vi "Simulation Kobuki Sensors.vi"(8 "error in":errorcluster, 9 "Feedback Input":T1, 10 "Robot":T2, 11 "simulator":T8={"configuration"={"maxTime"=5.0, "enableVisualization"=TRUE, "Environment Definition"=path "simulation configuration.ini", "Record Location"=path "Simulation Record.xml", "autograde?"=TRUE, "interactive?"=FALSE, "Feedback Mode"=enum."debug navigation", "Robot State Charts"=[path "C:/Users/blueuser/Desktop/Robo Sim Berkley/cpsgrader-release-0.4/Simulators/EECS149lab/src/LabVIEW/statechart/Simulation Statechart.vi"], "statechart"=path "iRobot Navigation State Machine.vi"}, "Statechart\ndisplay"=refnum, "first step?"=FALSE, "Robots Simulation Statecharts"=[], "Robots"=[]}) -> (0 "error out":errorcluster, 1 "Feedback Output":T1, 2 "sensors":T3 {"Kobuki Sensors"."Charger Source" items=["DISCHARGING"=0, "DOCKING_CHARGED"=2, "DOCKING_CHARGING"=6, "ADAPTER_CHARGED"=18, "ADAPTER_CHARGING"=22]; "accelerometer"."z axis (g)" format="%.3f"; "accelerometer"."y axis (g)" format="%.3f"; "accelerometer"."x axis (g)" format="%.3f"}, 3 "simulator":T8={"configuration"={"maxTime"=5.0, "enableVisualization"=TRUE, "Environment Definition"=path "simulation configuration.ini", "Record Location"=path "Simulation Record.xml", "autograde?"=TRUE, "interactive?"=FALSE, "Feedback Mode"=enum."debug navigation", "Robot State Charts"=[path "C:/Users/blueuser/Desktop/Robo Sim Berkley/cpsgrader-release-0.4/Simulators/EECS149lab/src/LabVIEW/statechart/Simulation Statechart.vi"], "statechart"=path "iRobot Navigation State Machine.vi"}, "Statechart\ndisplay"=refnum, "first step?"=FALSE, "Robots Simulation Statecharts"=[], "Robots"=[]})   [LabVIEW 2014]
doc: "Simulates iRobot sensors. Automatically accumulates distance and angle."
uses:
  Simulator.ctl
  <instrlib>/DC Motor Controller/HAIOL/DC Motor Controller.lvclass
  CyberSim interface/Simulation Configuration.ctl
  autograder/feedbackMode.ctl
  Multi Bot Code/RobotData.ctl
  shared/Sensors.ctl
  shared/Accelerometer.ctl
  Kobuki/KobukiSensors.ctl
  Kobuki/Kobuki Bumps and WheelDrops.ctl
  Kobuki/Kobuki Buttons.ctl
  Multi Bot Code/Sim Sensors Feedback.ctl
  <vilib>/Analysis/coordinate.llb/Angle Units.ctl
  <vilib>/Analysis/coordinate.llb/Wrap Angle (scalar).vi
  <vilib>/Analysis/BLAS.llb/dnrm2 - Vector 2-Norm (DBL).vi
  <resource>/objmgr/LVODE.rc
  <vilib>/Analysis/NI_AALBLAS.lvlib
  <vilib>/robotics/Kinematics/NI_Kinematics.lvlib
  <vilib>/Analysis/NI_AAL_Angle.lvlib
panel:
  out "Roll":dbl
  out "pitch":dbl
  out "Yaw":dbl
  # "Electrical: charging, battery, OI mode"
  # "Sensors: bump, cliff, button, wheel drop"
  # "Motors:"
  # "Inertia"
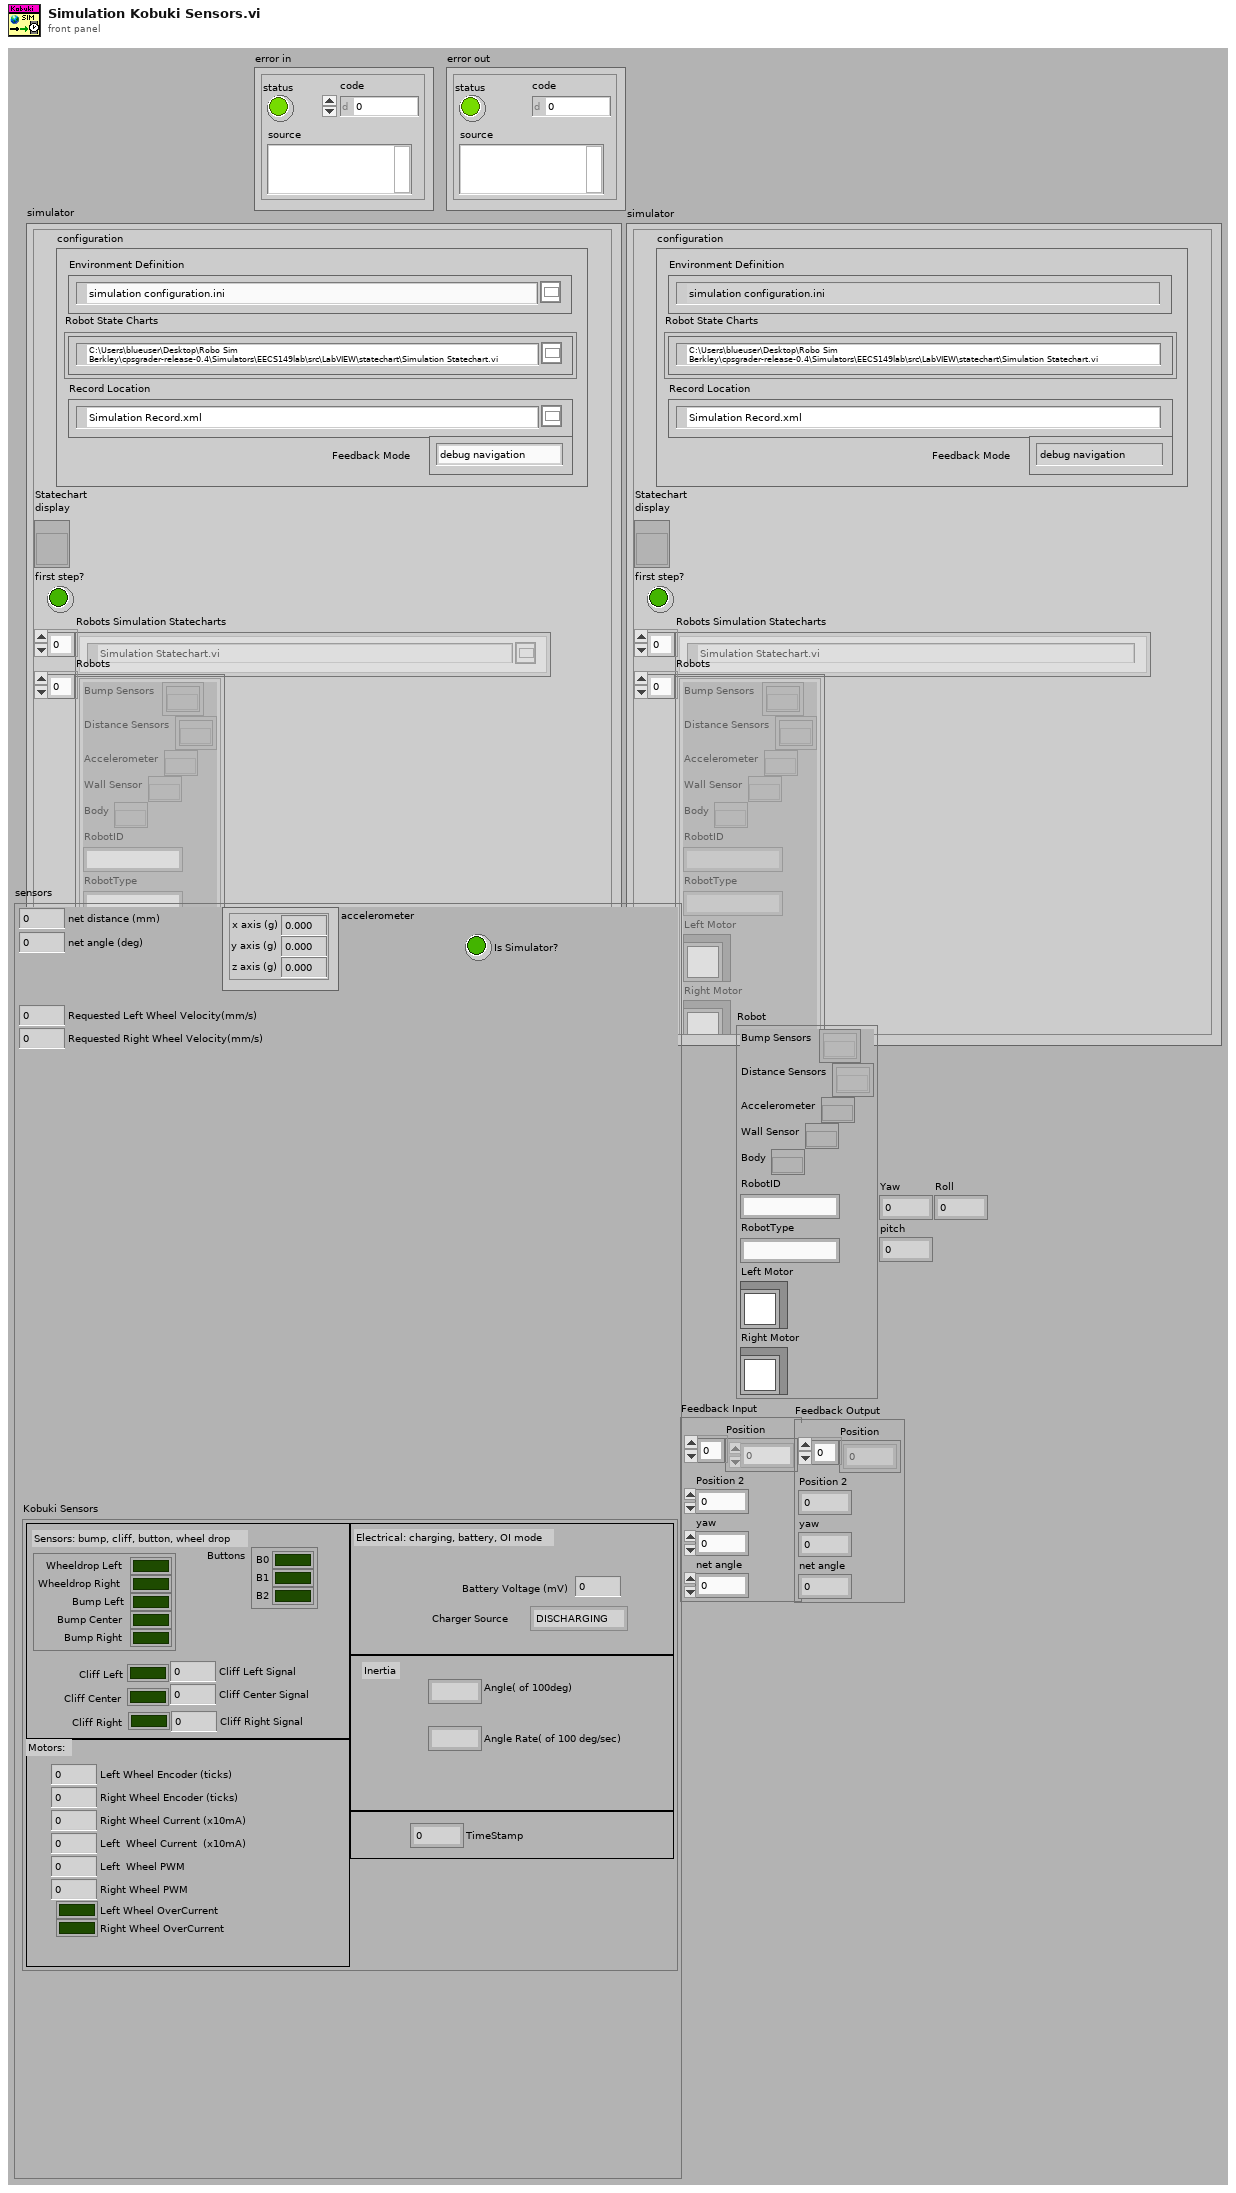
[diagram p1: front panel]
types:
  T1 = typedef "Sim Sensors Feedback.ctl" = cluster{"Position":sgl[], "Position 2":dbl, "yaw":dbl, "net angle":dbl}
  T2 = typedef "RobotData.ctl" = cluster{"Bump Sensors":refnum<k20>[], "Distance Sensors":refnum<k20>[], "Accelerometer":refnum<k20>, "Wall Sensor":refnum<k20>, "Body":refnum<k20>, "RobotID":string, "RobotType":string, "Left Motor":refnum<class "DC Motor Controller.lvclass">, "Right Motor":refnum<class "DC Motor Controller.lvclass">}
  T3 = typedef "Sensors.ctl" = cluster{"net distance (mm)":i32, "net angle (deg)":i32, "accelerometer":T4, "Is Simulator?":bool, "Kobuki Sensors":T5, "Requested Left Wheel Velocity(mm/s)":i32, "Requested Right Wheel Velocity(mm/s)":i32}
  T4 = typedef "Accelerometer.ctl" = cluster{"x axis (g)":dbl, "y axis (g)":dbl, "z axis (g)":dbl}
  T5 = typedef "KobukiSensors.ctl" = cluster{"Bumps + Wheel Drops":T6, "Cliff Left":bool, "Cliff Center":bool, "Cliff Right":bool, "Cliff Left Signal":u16, "Cliff Center Signal":u16, "Cliff Right Signal":u16, "Buttons":T7, "Left Wheel Encoder (ticks)":u16, "Right Wheel Encoder (ticks) ":u16, "Left  Wheel PWM":i8, "Right Wheel PWM":i8, "Left Wheel OverCurrent":bool, "Right Wheel OverCurrent ":bool, "Right Wheel Current (x10mA)":i16, "Left  Wheel Current  (x10mA)":i16, "TimeStamp":u16, "Battery Voltage (mV)":i16, "Angle( of 100deg)":i16, "Angle Rate( of 100 deg/sec)":i16, "Charger Source ":i8}
  T6 = typedef "Kobuki Bumps and WheelDrops.ctl" = cluster{"Wheeldrop Left":bool, "Wheeldrop Right":bool, "Bump Left":bool, "Bump Center":bool, "Bump Right":bool}
  T7 = typedef "Kobuki Buttons.ctl" = cluster{"B0":bool, "B1":bool, "B2":bool}
  T8 = typedef "Simulator.ctl" = cluster{"configuration":T9, "Statechart\ndisplay":refnum<vi>, "first step?":bool, "Robots Simulation Statecharts":path[], "Robots":T2[]}
  T9 = typedef "Simulation Configuration.ctl" = cluster{"maxTime":sgl, "enableVisualization":bool, "Environment Definition":path, "Record Location":path, "autograde?":bool, "interactive?":bool, "Feedback Mode":T10, "Robot State Charts":path[], "statechart":path}
  T10 = typedef "feedbackMode.ctl" = enum32{"debug navigation", "debug hill climb", "autograde navigation", "autograde hill climb"}
  T11 = typedef "NI_AAL_Angle.lvlib/Angle Units.ctl" = i32
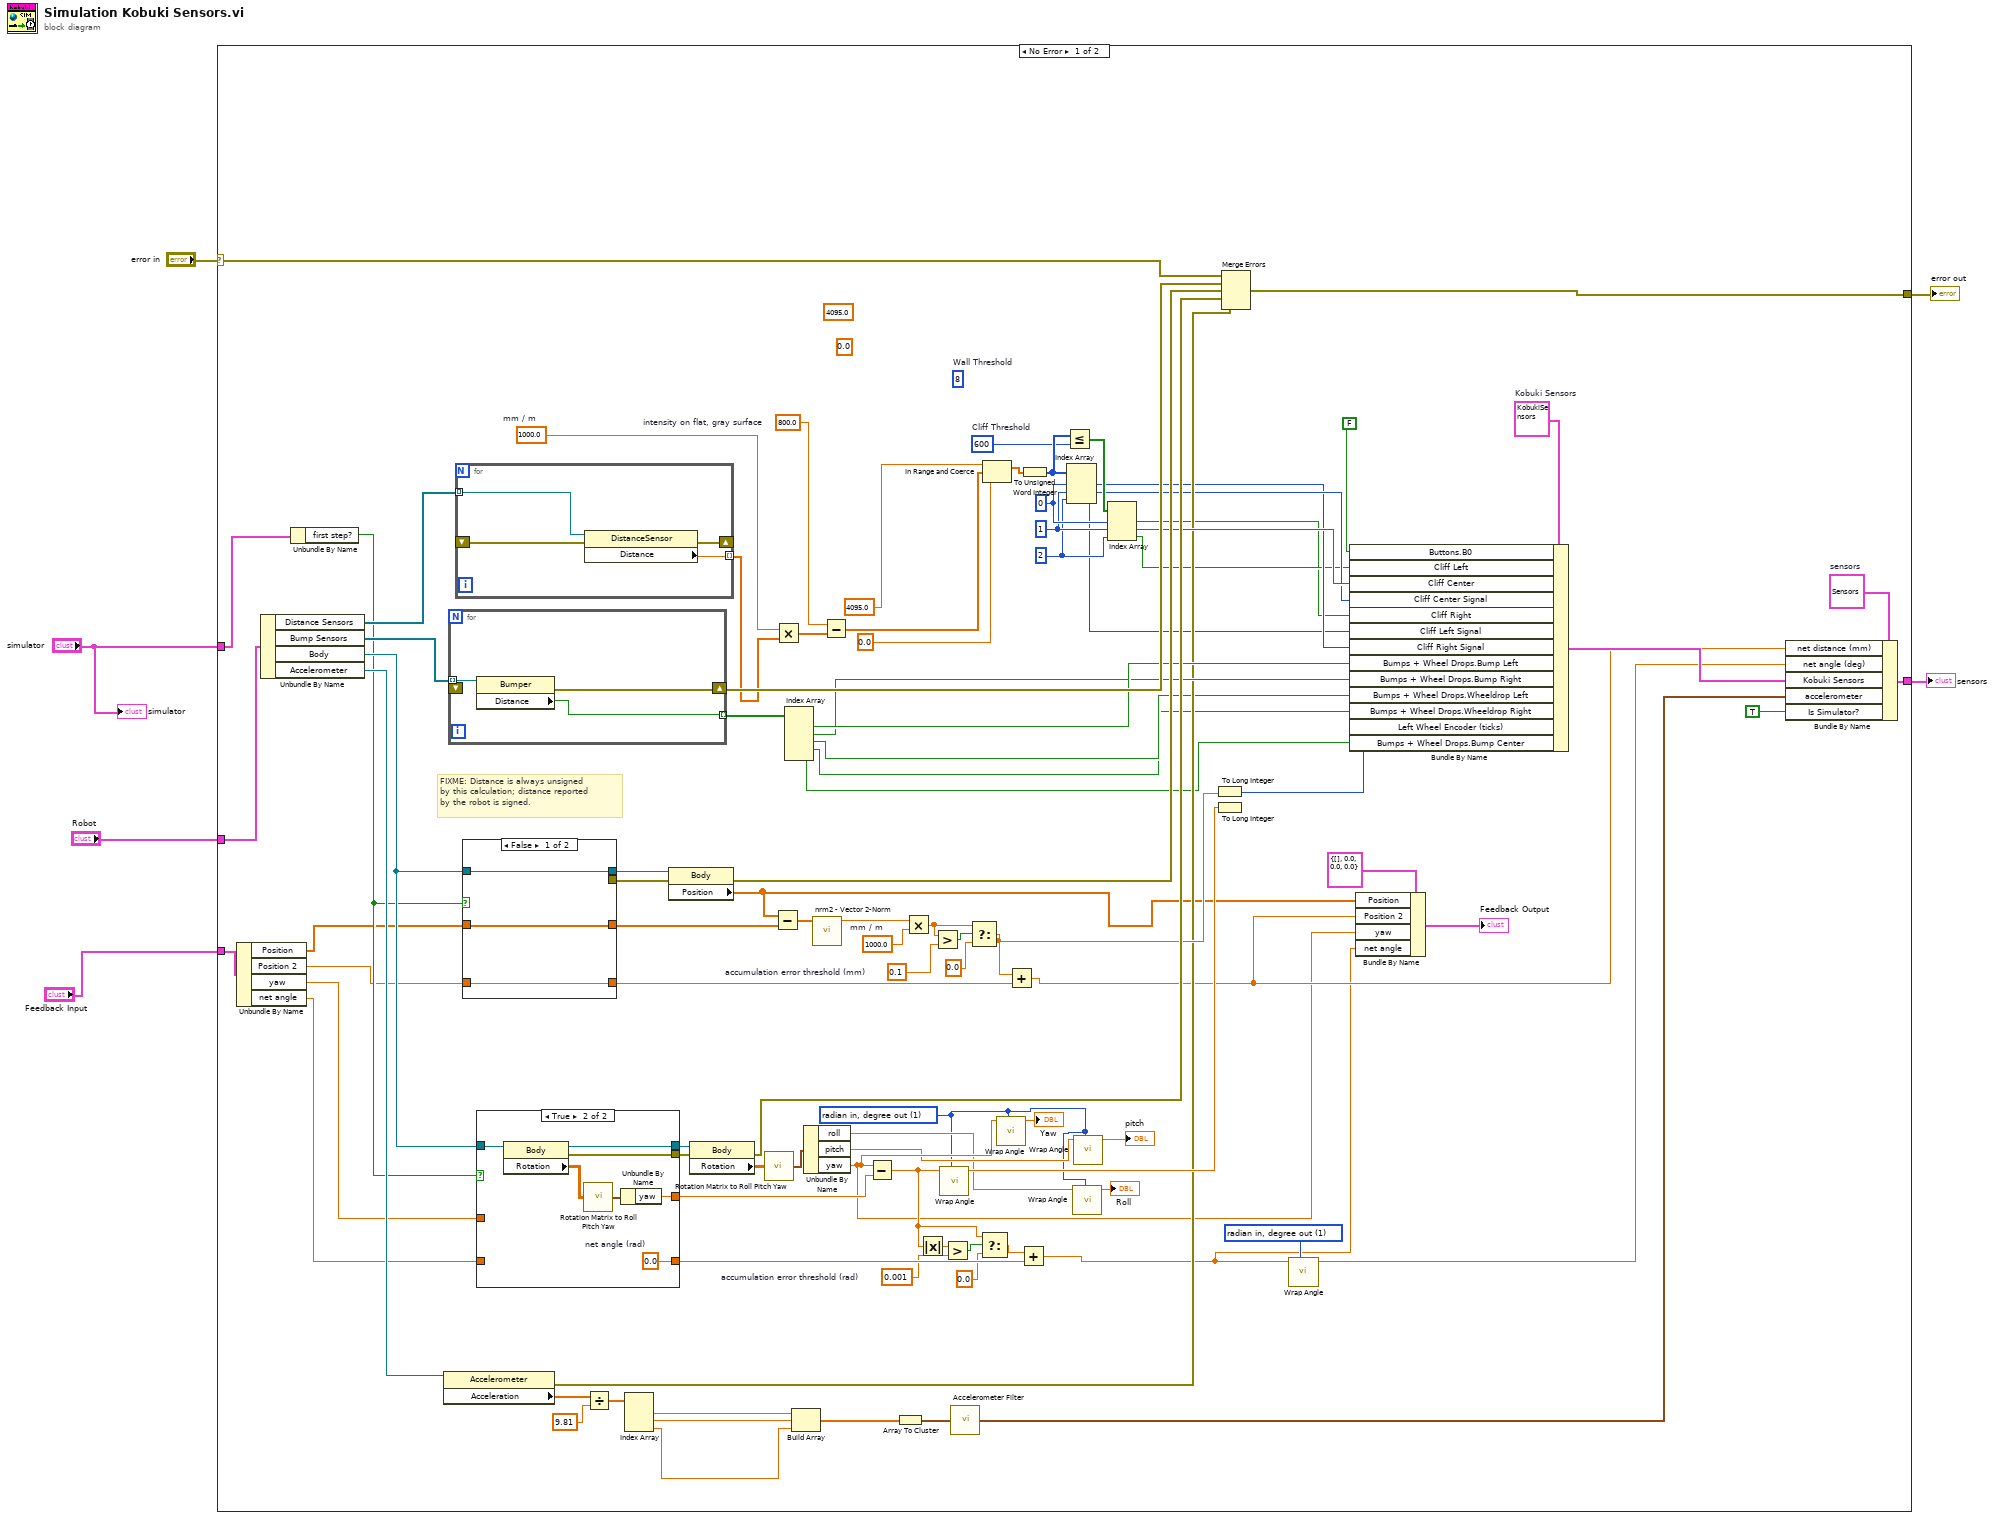
[diagram p0: block diagram]
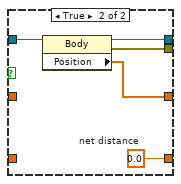
[diagram p3: hidden frame]
diagram:
  n1 = case shown="No Error" "error in" {
    selector: "error in" -> [w67 w131]
    tunnel: [w72 _] -> w6
    tunnel: "simulator" -> [w57 _]
    tunnel: [w68 w131] -> w4
    tunnel: "Robot" -> [w58 _]
    tunnel: "Feedback Input" -> [w55 _]
    frame No Error {
      w10 = T11 1 items=["radian in, radian out", "radian in, degree out", "degree in, degree out", "degree in, radian out"] ("angle units")
      w25 = 0.001  # accumulation error threshold (rad)
      w36 = 0.1  # accumulation error threshold (mm)
      w41 = 1000.0  # mm / m
      w20 = 2 ("index")
      w61 = 1 ("index")
      w62 = 0 ("index")
      w73 = T3 {"net distance (mm)"=0, "net angle (deg)"=0, "accelerometer"={"x axis (g)"=0.0, "y axis (g)"=0.0, "z axis (g)"=0.0}, "Is Simulator?"=FALSE, "Kobuki Sensors"={"Bumps + Wheel Drops"={"Wheeldrop Left"=FALSE, "Wheeldrop Right"=FALSE, "Bump Left"=FALSE, "Bump Center"=FALSE, "Bump Right"=FALSE}, "Cliff Left"=FALSE, "Cliff Center"=FALSE, "Cliff Right"=FALSE, "Cliff Left Signal"=0, "Cliff Center Signal"=0, "Cliff Right Signal"=0, "Buttons"={"B0"=FALSE, "B1"=FALSE, "B2"=FALSE}, "Left Wheel Encoder (ticks)"=0, "Right Wheel Encoder (ticks) "=0, "Left  Wheel PWM"=0, "Right Wheel PWM"=0, "Left Wheel OverCurrent"=FALSE, "Right Wheel OverCurrent "=FALSE, "Right Wheel Current (x10mA)"=0, "Left  Wheel Current  (x10mA)"=0, "TimeStamp"=0, "Battery Voltage (mV)"=0, "Angle( of 100deg)"=0, "Angle Rate( of 100 deg/sec)"=0, "Charger Source "=0}, "Requested Left Wheel Velocity(mm/s)"=0, "Requested Right Wheel Velocity(mm/s)"=0}  # sensors
      (unwired) 4095.0 ("upper limit")
      (unwired) 0.0 ("lower limit")
      (unwired) u16 8  # Wall Threshold
      w86 = 800.0  # intensity on flat, gray surface
      w89 = T11 1 items=["radian in, radian out", "radian in, degree out", "degree in, degree out", "degree in, radian out"] ("angle units")
      w90 = 600  # Cliff Threshold
      w99 = T5 {"Bumps + Wheel Drops"={"Wheeldrop Left"=FALSE, "Wheeldrop Right"=FALSE, "Bump Left"=FALSE, "Bump Center"=FALSE, "Bump Right"=FALSE}, "Cliff Left"=FALSE, "Cliff Center"=FALSE, "Cliff Right"=FALSE, "Cliff Left Signal"=0, "Cliff Center Signal"=0, "Cliff Right Signal"=0, "Buttons"={"B0"=FALSE, "B1"=FALSE, "B2"=FALSE}, "Left Wheel Encoder (ticks)"=0, "Right Wheel Encoder (ticks) "=0, "Left  Wheel PWM"=0, "Right Wheel PWM"=0, "Left Wheel OverCurrent"=FALSE, "Right Wheel OverCurrent "=FALSE, "Right Wheel Current (x10mA)"=0, "Left  Wheel Current  (x10mA)"=0, "TimeStamp"=0, "Battery Voltage (mV)"=0, "Angle( of 100deg)"=0, "Angle Rate( of 100 deg/sec)"=0, "Charger Source "=0}  # Kobuki Sensors
      w103 = 1000.0  # mm / m
      # "FIXME: Distance is always unsigned\nby this calculation; distance reported\nby the robot is signed."
      n2 = Unbundle By Name(w55) -> ("Position"=w54:sgl[], "Position 2"=w53:dbl, "yaw"=w52:dbl, "net angle"=w51:dbl)
      n3 = Unbundle By Name(w58) -> ("Distance Sensors"=w64:refnum<k20>[], "Bump Sensors"=w105:refnum<k20>[], "Body"=w88:refnum<k20>, "Accelerometer"=w81:refnum<k20>)
      n4 = Unbundle By Name(w57) -> ("first step?"=w56:bool)
      n5 = property class="Accelerometer"(reference=w81) -> (error out=w66:errorcluster, "Acceleration"=w80:sgl[])  [unwired: 1 in, 1 out]
      n6 = for {
        tunnel: w105 -> [w130] mode=indexing
        tunnel: [w129] -> w104 mode=indexing
        shift-right: [w128] -> w102
        shift-left: _ -> [_]
        n7 = property class="Bumper"(reference=w130) -> (error out=w128:errorcluster, "Distance"=w129:bool)  [unwired: 1 in, 1 out]
      }
      n8 = for {
        tunnel: [w127] -> w63 mode=indexing
        shift-right: [w126] -> _
        shift-left: _ -> [w124]
        tunnel: w64 -> [w125] mode=indexing
        n9 = property class="DistanceSensor"(reference=w125, error in=w124) -> (error out=w126:errorcluster, "Distance"=w127:sgl)  [unwired: 1 out]
      }
      n10 = case shown="False" w56 {
        tunnel: w88 -> [w117 w123]
        tunnel: [w118 w120] -> w43
        tunnel: w54 -> [w118 _]
        tunnel: [_ w122] -> w44
        tunnel: [w117 w121] -> w45
        tunnel: w53 -> [w116 _]
        tunnel: [w116 w119] -> w39
        frame False {
        }
        frame True {
          w119 = 0.0  # net distance
          n11 = property class="Body"(reference=w123) -> (reference out=w121:refnum<k20>, error out=w122:errorcluster, "Position"=w120:sgl[])  [unwired: 1 in]
        }
      }
      n12 = case shown="True" w56 {
        tunnel: w88 -> [w108 w115]
        tunnel: [w108 w114] -> w34
        tunnel: [_ w113] -> w33
        tunnel: [w107 w110] -> w30
        tunnel: w52 -> [w107 _]
        tunnel: [w106 w109] -> w27
        tunnel: w51 -> [w106 _]
        frame False {
        }
        frame True {
          w109 = 0.0  # net angle (rad)
          n13 = property class="Body"(reference=w115) -> (reference out=w114:refnum<k20>, error out=w113:errorcluster, "Rotation"=w112:sgl[][])  [unwired: 1 in]
          n14 = call <vilib>:"Rotation Matrix to Roll Pitch Yaw.vi"("rotation matrix"=w112) -> ("angles"=w111:cluster{"roll":dbl, "pitch":dbl, "yaw":dbl})
          n15 = Unbundle By Name(w111) -> ("yaw"=w110:dbl)
        }
      }
      n16 = Divide(x=w80, y=9.81) -> (x/y=w78:dbl[])
      n17 = Index Array(array=w78) -> (element #1=w8:dbl, element #2=w7:dbl, element #3=w77:dbl)  [unwired: 3 in]
      n18 = property class="Body"(reference=w45, error in=w44) -> (error out=w101:errorcluster, "Position"=w48:sgl[])  [unwired: 1 out]
      n19 = property class="Body"(reference=w34, error in=w33) -> (error out=w100:errorcluster, "Rotation"=w32:sgl[][])  [unwired: 1 out]
      n20 = call <vilib>:"Rotation Matrix to Roll Pitch Yaw.vi"("rotation matrix"=w32) -> ("angles"=w31:cluster{"roll":dbl, "pitch":dbl, "yaw":dbl})
      n21 = Subtract(x=w48, y=w43) -> (x-y=w40:sgl[])
      n22 = Multiply(x=w103, y=w63) -> (x*y=w87:dbl[])
      n23 = Index Array(array=w104) -> (element #1=w98:bool, element #2=w97:bool, element #3=w22:bool, element #4=w21:bool, element #5=w59:bool)  [unwired: 5 in]
      n24 = Build Array(w8, w7, w77) -> (w76:dbl[])
      n25 = Unbundle By Name(w31) -> ("roll"=w11:dbl, "pitch"=w13:dbl, "yaw"=w15:dbl)
      n26 = call-poly <vilib>:"nrm2 - Vector 2-Norm.vi"("x"=w40) -> ("dnrm2"=w42:dbl)  [unwired: 9 in, 1 out]
      n27 = Subtract(x=w86, y=w87) -> (x-y=w83:dbl[])
      n28 = Subtract(x=w15, y=w30) -> (x-y=w23:dbl)
      n29 = Array To Cluster(array=w76) -> (cluster=w70:cluster{"[0]":dbl, "[1]":dbl, "[2]":dbl})
      n30 = Multiply(x=w42, y=w41) -> (x*y=w38:dbl)
      n31 = Absolute Value(x=w23) -> (abs(x)=w24:dbl)
      n32 = Greater?(x=w38, y=w36) -> (0:w37:bool)
      n33 = call-poly <vilib>:"Wrap Angle.vi"("angle units"=w10, "angle in"=w23) -> ("angle out"=w94:dbl)  [unwired: 8 in, 1 out]
      n34 = Greater?(x=w24, y=w25) -> (0:w29:bool)
      n35 = call "Accelerometer Filter.vi"("accelerometer (g)"=w70) -> ("filtered accelerometer (g)"=w69:T4)  [unwired: 3 in]
      n36 = Select(t=w38, s=w37, f=0.0) -> (s? t:f=w95:dbl)
      n37 = Select(t=w23, s=w29, f=0.0) -> (s? t:f=w28:dbl)
      n38 = In Range and Coerce(upper limit=4095.0, x=w83, lower limit=0.0) -> (coerced(x)=w82:dbl[])  [unwired: 1 out]
      n39 = call-poly <vilib>:"Wrap Angle.vi"("angle units"=w10, "angle in"=w15) -> ("angle out"=→"Yaw":dbl)  [unwired: 8 in, 1 out]
      n40 = Add(x=w95, y=w39) -> (x+y=w47:dbl)
      n41 = Add(x=w28, y=w27) -> (x+y=w46:dbl)
      n42 = To Unsigned Word Integer(number=w82) -> (unsigned 16bit integer=w93:u16[])
      n43 = Less Or Equal?(x=w93, y=w90) -> (x <= y?=w92:bool[])
      n44 = Index Array(array=w93, index #1=w62, index #2=w61, index #3=w20) -> (element #1=w19:u16, element #2=w60:u16, element #3=w18:u16)
      n45 = call-poly <vilib>:"Wrap Angle.vi"("angle units"=w10, "angle in"=w11) -> ("angle out"=→"Roll":dbl)  [unwired: 8 in, 1 out]
      n46 = call-poly <vilib>:"Wrap Angle.vi"("angle units"=w10, "angle in"=w13) -> ("angle out"=→"pitch":dbl)  [unwired: 8 in, 1 out]
      n47 = Index Array(array=w92, index #1=w62, index #2=w61, index #3=w20) -> (element #1=w16:bool, element #2=w91:bool, element #3=w17:bool)
      n48 = To Long Integer(number=w95) -> (32bit integer=w96:i32)
      n49 = To Long Integer(number=w94) -> ()  [unwired: 1 out]
      n50 = Merge Errors(w67, w102, w101, w100, w66) -> (w68:errorcluster)
      n51 = call-poly <vilib>:"Wrap Angle.vi"("angle units"=w89, "angle in"=w46) -> ("angle out"=w74:dbl)  [unwired: 8 in, 1 out]
      n52 = Bundle By Name(cluster=w99, "Buttons.B0"=FALSE ("Buttons.Play"), "Cliff Left"=w17, "Cliff Center"=w91, "Cliff Center Signal"=w60, "Cliff Right"=w16, "Cliff Left Signal"=w18, "Cliff Right Signal"=w19, "Bumps + Wheel Drops.Bump Left"=w98, "Bumps + Wheel Drops.Bump Right"=w97, "Bumps + Wheel Drops.Wheeldrop Left"=w22, "Bumps + Wheel Drops.Wheeldrop Right"=w21, "Left Wheel Encoder (ticks)"=w96, "Bumps + Wheel Drops.Bump Center"=w59) -> (w75:T5)
      n53 = Bundle By Name(cluster=T1 {"Position"=[], "Position 2"=0.0, "yaw"=0.0, "net angle"=0.0} ("output cluster"), "Position"=w48, "Position 2"=w47, "yaw"=w15, "net angle"=w46) -> (→"Feedback Output":T1)
      n54 = Bundle By Name(cluster=w73, "net distance (mm)"=w47, "net angle (deg)"=w74, "Kobuki Sensors"=w75, "accelerometer"=w69, "Is Simulator?"=TRUE) -> (w72:T3)
    }
    frame Error {
    }
  }
  "error out" <- w4
  "sensors" <- w6
  "simulator" <- "simulator"
